vi "Generate Running Averages By Factor of 10.vi"(11 "Input":dbl[](array[numeric])) -> (3 "Averages":dbl[][](array[numeric]))   [LabVIEW 2018]
uses:
  <vilib>/ptbypt/NI_PtbyPt.lvlib
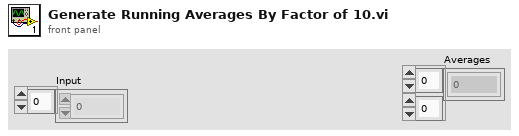
[diagram p1: front panel]
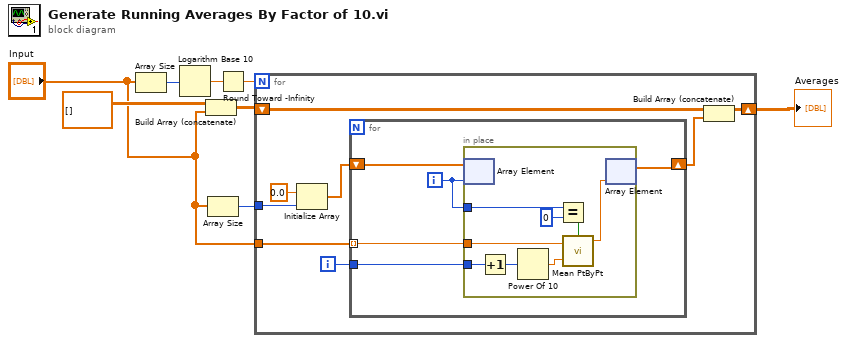
[diagram p0: block diagram]
diagram:
  n1 = Array Size(array="Input") -> (size(s)=w8:i32)
  n2 = Logarithm Base 10(1:w8) -> (0:w7:dbl)
  n3 = Build Array (concatenate)(dbl[][] [], "Input") -> (w4:dbl[][])
  n4 = Array Size(array="Input") -> (size(s)=w6:i32)
  n5 = Round Toward -Infinity(1:w7) -> (0:w5:dbl)
  n6 = for {
    N: w5 -> [_]
    tunnel: w6 -> [w16]
    tunnel: "Input" -> [w13]
    shift-right: [w11] -> w1
    shift-left: w4 -> [w9]
    i -> [w12]
    n7 = Initialize Array(0.0 ("element"), w16) -> (w14:dbl[])
    n8 = for {
      shift-right: [w20] -> w10
      shift-left: w14 -> [w21]
      tunnel: w13 -> [w19] mode=indexing
      tunnel: w12 -> [w17]
      i -> [w18]
      n9 = in-place {
        in-place-border: w19 -> [w25]
        in-place-border: w18 -> [w24]
        in-place-border: w17 -> [w23]
        n10 = in-place-array #1(w21, w18) -> ()  [unwired: 1 out]
        n11 = Increment(x=w23) -> (x+1=w28:i32)
        n12 = Power Of 10(x=w28) -> (10^x=w29:dbl)
        n13 = Equal?(x=w24, y=0) -> (x = y?=w26:bool)
        n14 = call <vilib>:"Mean PtByPt.vi"("x"=w25, "sample length"=w29, "initialize"=w26) -> ("mean"=w22:dbl)  [unwired: 1 in, 1 out]
        n15 = in-place-array #1(w22) -> (w20:dbl[])  [unwired: 1 out]
      }
    }
    n16 = Build Array (concatenate)(w9, w10) -> (w11:dbl[][])
  }
  "Averages" <- w1
